vi "_toString.vi"(8 "error in (no error)":errorcluster, 11 "CalibReport in":refnum<class "CalibReport.lvclass">) -> (0 "error out":errorcluster, 2 "<JSON>":string, 3 "CalibReport out":refnum<class "CalibReport.lvclass">)   [LabVIEW 2024, in "CalibReport.lvclass"]
uses:
  CalibReport.lvclass
  CalibReport.lvclass/CalibReport.ctl
  b2739898-71ad-4109-afcf-259c3fe9574e.vi
  b3db79ce-2d40-4964-941b-d0bca1e08292.vi
  38357d63-789c-4284-b7e5-e7d0e442af8b.vi
  <vilib>/JDP Science/JSONtext/Variant to JSON Text.vi
  <vilib>/JDP Science/JSONtext/support/Format JSON Array Text.vi
  <vilib>/JDP Science/JSONtext/support/Format JSON Object.vi
  <vilib>/JDP Science/JSONtext/LVClass Serializer/JSONtext LVClass Serializer.lvclass
  <vilib>/JDP Science/JSONtext/JSONtext.lvlib
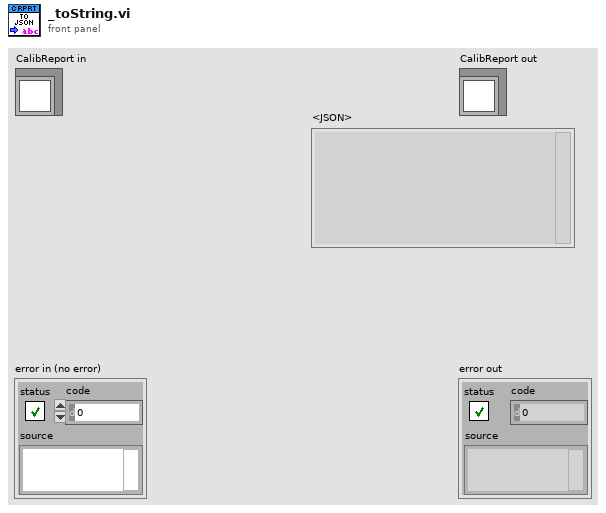
[diagram p1: front panel]
types:
  T1 = typedef "cReportEntry.ctl" = cluster{"Reference [kg]":dbl, "DUT value [kg]":dbl}
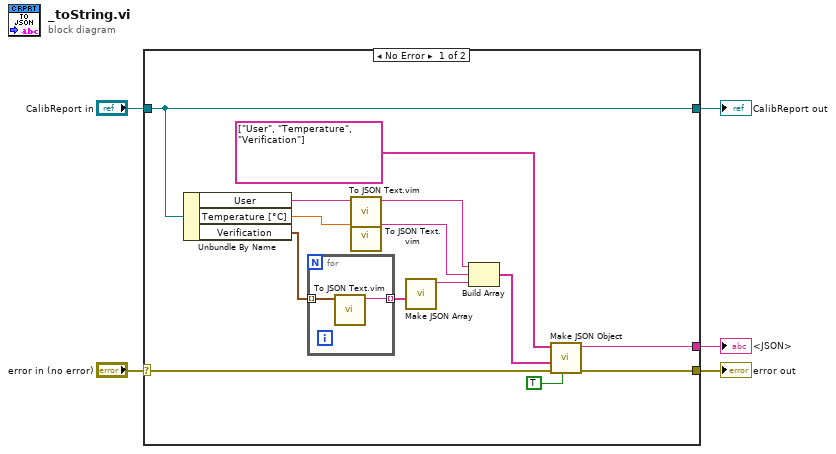
[diagram p0: block diagram]
diagram:
  n1 = case shown="No Error" "error in (no error)" {
    selector: "error in (no error)" -> [w16 w23]
    tunnel: [w15 w23] -> w4
    tunnel: [w19 w22] -> w2
    tunnel: "CalibReport in" -> [w19 w22]
    tunnel: [w7 _] -> w1
    frame No Error {
      n2 = Unbundle By Name(w19) -> ("User"=w18:string, "Temperature [°C]"=w17:dbl, "Verification"=w13:T1[])
      n3 = for {
        tunnel: w13 -> [w21] mode=indexing
        tunnel: [w20] -> w12 mode=indexing
        n4 = call "To JSON Text.vim"("Anything"=w21) -> ("<JSON>"=w20:string)  [unwired: 9 in, 1 out]
      }
      n5 = call "To JSON Text.vim"("Anything"=w18) -> ("<JSON>"=w11:string)  [unwired: 9 in, 1 out]
      n6 = call "To JSON Text.vim"("Anything"=w17) -> ("<JSON>"=w10:string)  [unwired: 9 in, 1 out]
      n7 = call <vilib>:"Make JSON Array.vi"("JSON Elements"=w12) -> ("<JSON>"=w9:string)  [unwired: 9 in, 1 out]
      n8 = Build Array(w11, w10, w9) -> (w8:string[])
      n9 = call <vilib>:"Make JSON Object.vi"("Pretty Print?"=TRUE, "error in (no error)"=w16, "JSON Items"=w8, "Item Names"=string[] ["User", "Temperature", "Verification"]) -> ("error out"=w15:errorcluster, "<JSON>"=w7:string)  [unwired: 6 in]
    }
    frame Error {
    }
  }
  "error out" <- w4
  "CalibReport out" <- w2
  "<JSON>" <- w1
